vi "RaiseArm.vi"(8 "error in":errorcluster, 9 "FPGA VI Reference In":T1, 10 "milliseconds to wait \nfor servo to change":u32=100, 11 "Old Angle":dbl) -> (0 "error out":errorcluster, 1 "FPGA VI Reference Out 2":T1, 2 "milliseconds to wait \nfor servo to change Out":u32, 3 "New Angle":dbl)   [LabVIEW 2012]
uses:
  FPGA_ref.ctl
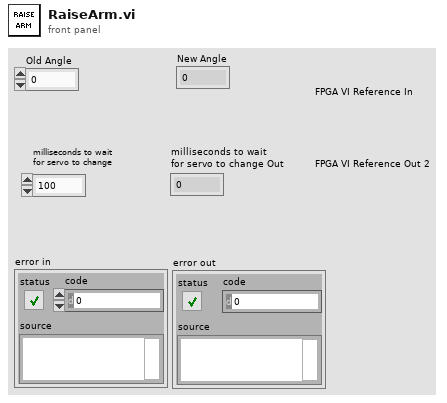
[diagram p1: front panel]
types:
  T1 = typedef "FPGA_ref.ctl" = refnum<k20>
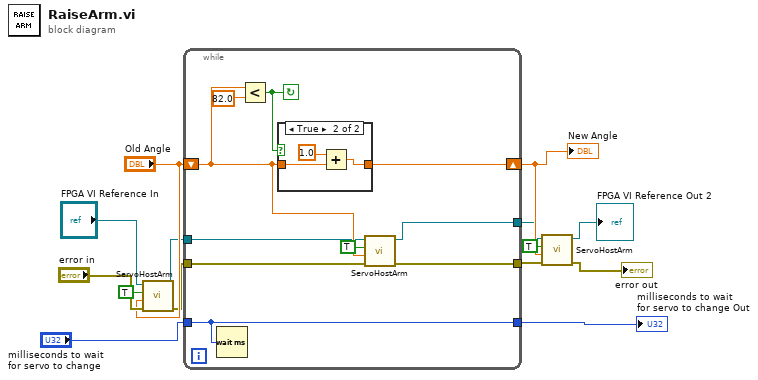
[diagram p0: block diagram]
diagram:
  n1 = call "ServoHostArm.vi"("error in"="error in", "Angle (deg) Arm"="Old Angle", "Enable"=TRUE, "FPGA VI Reference In"="FPGA VI Reference In") -> ("error out"=w7:errorcluster, "FPGA VI Reference Out 2"=w8:T1)  [unwired: 6 in]
  n2 = while {
    tunnel: w7 -> [w24]
    shift-right: [w20] -> w6
    shift-left: "Old Angle" -> [w21]
    tunnel: "milliseconds to wait \nfor servo to change" -> [w18]
    tunnel: [w19] -> w3
    tunnel: [w18] -> w14
    tunnel: w8 -> [w17]
    tunnel: [w16] -> w5
    stop <- w22 continue-if-true
    n3 = Wait (ms)(milliseconds to wait=w18) -> ()  [unwired: 1 out]
    n4 = Less?(x=w21, y=82.0) -> (x < y?=w22:bool)
    n5 = case shown="True" w22 {
      tunnel: w21 -> [w25 w28]
      tunnel: [w25 w26] -> w20
      frame False {
      }
      frame True {
        n6 = Add(x=1.0, y=w28) -> (x+y=w26:dbl)
      }
    }
    n7 = call "ServoHostArm.vi"("error in"=w24, "Angle (deg) Arm"=w21, "Enable"=TRUE, "FPGA VI Reference In"=w17) -> ("error out"=w19:errorcluster, "FPGA VI Reference Out 2"=w16:T1)  [unwired: 6 in]
  }
  "New Angle" <- w6
  "milliseconds to wait \nfor servo to change Out" <- w14
  n8 = call "ServoHostArm.vi"("error in"=w3, "Angle (deg) Arm"=w6, "Enable"=TRUE, "FPGA VI Reference In"=w5) -> ("error out"=→"error out":errorcluster, "FPGA VI Reference Out 2"=→"FPGA VI Reference Out 2":T1)  [unwired: 6 in]
